vi "SDO download (array).vi"(4 "Value":u8[](array[numeric]), 5 "Wait?":bool, 6 "error in (no error)":errorcluster, 7 "Multiplexor":T1 {"Sub-index" format="%02x"; "Index" format="%04x"}, 8 "Node ID":u8, 9 "CANopen in":refnum<class "CANopen.lvclass">) -> (0 "error out":errorcluster, 3 "CANopen out":refnum<class "CANopen.lvclass">)   [LabVIEW 2017, in "canopen.lvlib" / "CANopen.lvclass"]
doc: "Writes a value in the open dictionary of a CANopen node."
uses:
  CANopen.lvclass
  Multiplexor.ctl
  FunctionCode.ctl
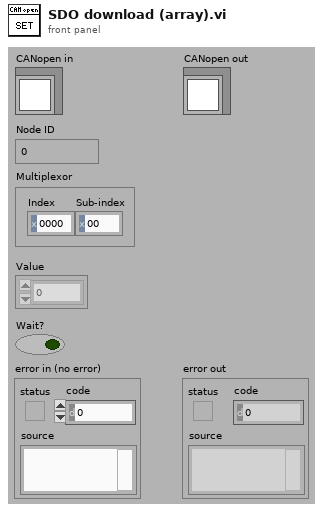
[diagram p1: front panel]
types:
  T1 = typedef "canopen.lvlib/CANopen.lvclass/Multiplexor.ctl" = cluster{"Index":u16, "Sub-index":u8}
  T2 = typedef "canopen.lvlib/CANopen.lvclass/FunctionCode.ctl" = u8
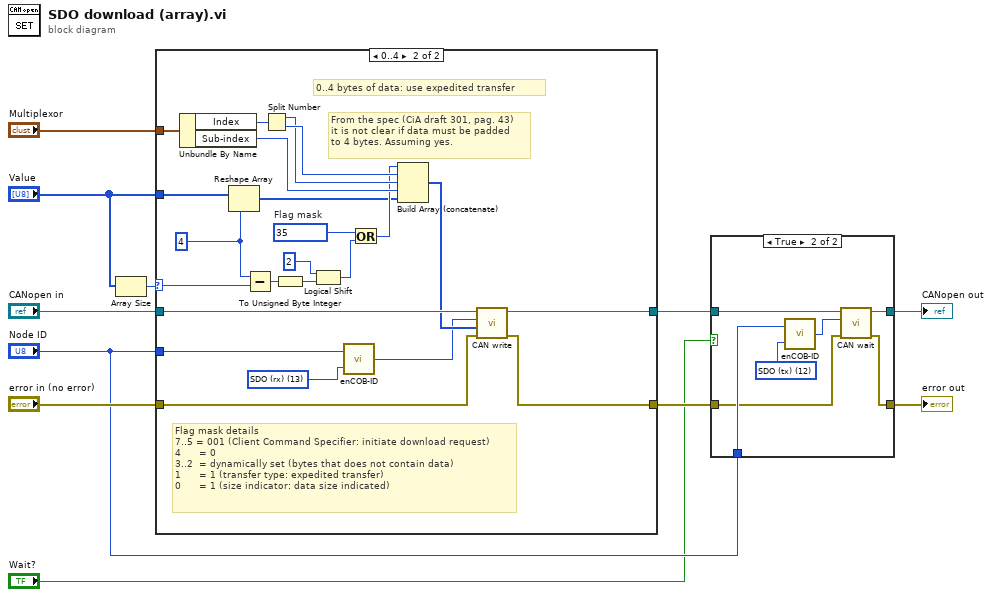
[diagram p0: block diagram]
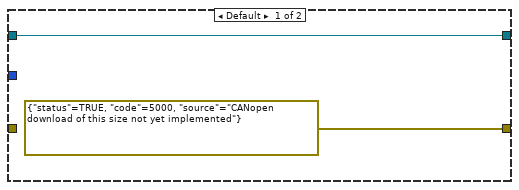
[diagram p3: hidden frame]
diagram:
  n1 = Array Size(array="Value") -> (size(s)=w10:i32)
  n2 = case shown="0..4" w10 {
    selector: w10 -> [_ w21]
    tunnel: "CANopen in" -> [w13 w36]
    tunnel: [w13 w35] -> w6
    tunnel: [errorcluster {"status"=TRUE, "code"=5000, "source"="CANopen download of this size not yet implemented"} ("error out") w34] -> w2
    tunnel: "Node ID" -> [_ w15]
    tunnel: "error in (no error)" -> [_ w17]
    tunnel: "Value" -> [_ w25]
    tunnel: "Multiplexor" -> [_ w33]
    frame Default {
    }
    frame 0..4 {
      w18 = T2 13 items=["NMT", "SYNC", "TIME STAMP", "EMERGENCY", "PDO1 (tx)", "PDO1 (rx)", "PDO2 (tx)", "PDO2 (rx)", "PDO3 (tx)", "PDO3 (rx)", "PDO4 (tx)", "PDO4 (rx)", "SDO (tx)", "SDO (rx)", "NMT Error Control"] ("Function code")
      w26 = u8 35  # Flag mask
      w23 = 4 ("y")
      # "From the spec (CiA draft 301, pag. 43)\nit is not clear if data must be padded\nto 4 bytes. Assuming yes."
      # "Flag mask details\n7..5 = 001 (Client Command Specifier: initiate download request)\n4      = 0\n3..2  = dynamically set (bytes that does not contain data)\n1      = 1 (transfer type: expedited transfer)\n0      = 1 (size indicator: data size indicated)"
      # "0..4 bytes of data: use expedited transfer"
      n3 = Unbundle By Name(w33) -> ("Index"=w32:u16, "Sub-index"=w29:u8)
      n4 = Reshape Array(w25, w23) -> (w24:u8[])
      n5 = Subtract(x=w23, y=w21) -> (x-y=w22:i32)
      n6 = Split Number(x=w32) -> (hi(x)=w30:u8, lo(x)=w31:u8)
      n7 = To Unsigned Byte Integer(number=w22) -> (unsigned 8bit integer=w20:u8)
      n8 = Logical Shift(y=i8 2, x=w20) -> (x << y=w19:u8)
      n9 = call "enCOB-ID.vi"("Function code"=w18, "Node ID"=w15) -> ("Cob ID"=w14:u32)
      n10 = Or(x=w26, y=w19) -> (x .or. y?=w27:u8)
      n11 = Build Array (concatenate)(w27, w31, w30, w29, w24) -> (w16:u8[])
      n12 = call "CAN write.vi"("error in (no error)"=w17, "Data"=w16, "COB id"=w14, "CANopen in"=w36) -> ("error out"=w34:errorcluster, "CANopen out"=w35:refnum<class "CANopen.lvclass">)  [unwired: 1 in, 1 out]
    }
  }
  n13 = case shown="True" "Wait?" {
    tunnel: w6 -> [w38 w44]
    tunnel: [w38 w43] -> w5
    tunnel: "Node ID" -> [_ w42]
    tunnel: [w37 w41] -> w3
    tunnel: w2 -> [w37 w40]
    frame False {
    }
    frame True {
      w45 = T2 12 items=["NMT", "SYNC", "TIME STAMP", "EMERGENCY", "PDO1 (tx)", "PDO1 (rx)", "PDO2 (tx)", "PDO2 (rx)", "PDO3 (tx)", "PDO3 (rx)", "PDO4 (tx)", "PDO4 (rx)", "SDO (tx)", "SDO (rx)", "NMT Error Control"] ("Function code")
      n14 = call "enCOB-ID.vi"("Function code"=w45, "Node ID"=w42) -> ("Cob ID"=w39:u32)
      n15 = call "CAN wait.vi"("error in (no error)"=w40, "Cob ID"=w39, "CANopen in"=w44) -> ("error out"=w41:errorcluster, "CANopen out"=w43:refnum<class "CANopen.lvclass">)  [unwired: 1 in, 2 out]
    }
  }
  "error out" <- w3
  "CANopen out" <- w5
